vi "selfConfigRead.vi"(0 "RefDesType":string, 5 "error in":errorcluster) -> (14 "DAQ Node Array":string[](array[string]), 15 "DAQ Node Count":i32, 16 "refDes":string, 17 "IPaddr":string, 19 "error out":errorcluster)   [LabVIEW 2024]
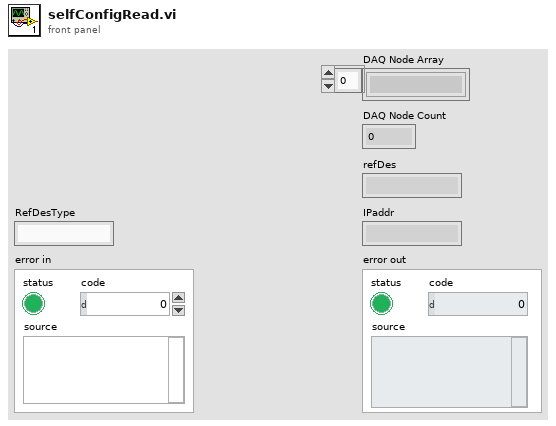
[diagram p1: front panel]
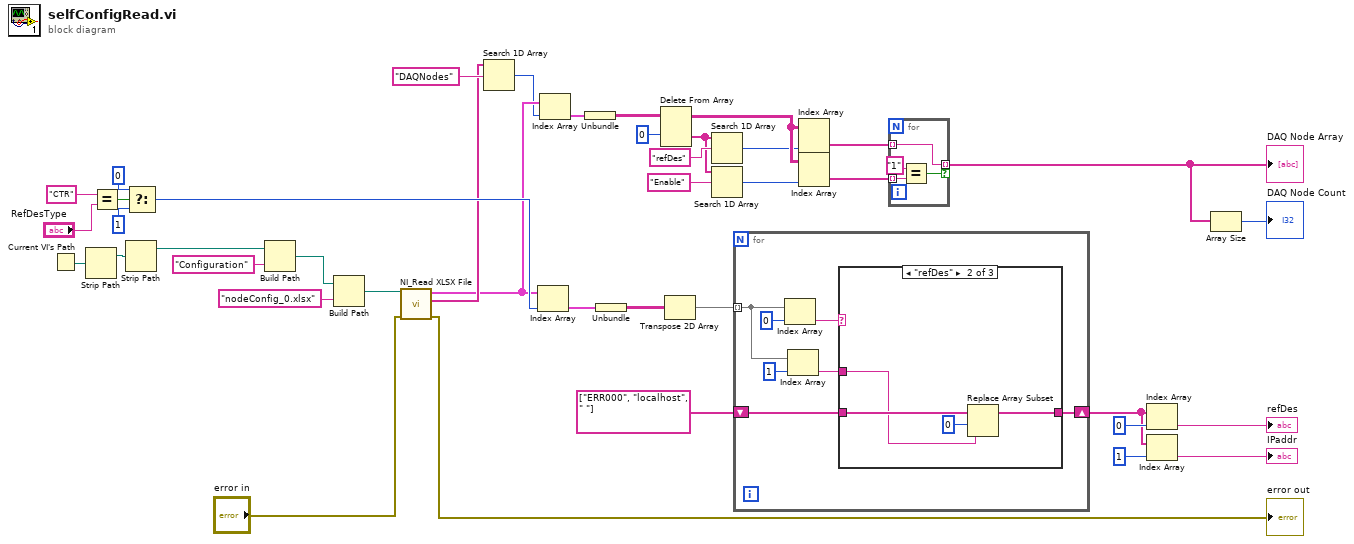
[diagram p0: block diagram]
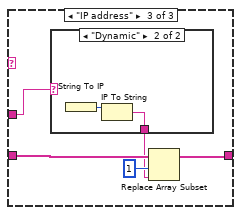
[diagram p3: hidden frame]
diagram:
  n1 = Current VI's Path() -> (path=w39:path)
  n2 = Strip Path(path=w39) -> (stripped path=w31:path)  [unwired: 1 out]
  n3 = Equal?(x="CTR", y="RefDesType") -> (x = y?=w27:bool)
  n4 = Strip Path(path=w31) -> (stripped path=w30:path)  [unwired: 1 out]
  n5 = Select(t=0, s=w27, f=1) -> (s? t:f=w24:i32)
  n6 = Build Path(base path=w30, name or relative path="Configuration") -> (appended path=w32:path)
  n7 = Build Path(base path=w32, name or relative path="nodeConfig_0.xlsx") -> (appended path=w40:path)
  n8 = call "NI_Read XLSX File.vi"("error in"="error in", "XLSX File"=w40) -> ("error out"=→"error out":errorcluster, "Sheet Names"=w16:string[], "Sheet Data"=w15:cluster{"Array":string[][]}[])  [unwired: 7 in]
  n9 = Search 1D Array(1D array=w16, element="DAQNodes") -> (index of element=w14:i32)  [unwired: 1 in]
  n10 = Index Array(array=w15, index=w24) -> (element=w23:cluster{"Array":string[][]})
  n11 = Index Array(array=w15, index=w14) -> (element=w13:cluster{"Array":string[][]})
  n12 = Unbundle(w13) -> ("Array"=w9:string[][])
  n13 = Unbundle(w23) -> ("Array"=w22:string[][])
  n14 = Delete From Array(array=w9, index (row)=0) -> (deleted portion=w8:string[], array with subset deleted=w7:string[][])  [unwired: 2 in]
  n15 = Transpose 2D Array(2D array=w22) -> (transposed array=w21:string[][])
  n16 = Search 1D Array(1D array=w8, element="refDes") -> (index of element=w5:i32)  [unwired: 1 in]
  n17 = Search 1D Array(1D array=w8, element="Enable") -> (index of element=w6:i32)  [unwired: 1 in]
  n18 = for {
    tunnel: w21 -> [w46] mode=indexing
    shift-right: [w43] -> w19
    shift-left: string[] ["ERR000", "localhost", " "] -> [w44]
    n19 = Index Array(array=w46, index=0) -> (element=w45:string)
    n20 = Index Array(array=w46, index=1) -> (element=w42:string)
    n21 = case shown="\"refDes\"" w45 {
      tunnel: w44 -> [w49 w53 w57]
      tunnel: [w49 w52 w56] -> w43
      tunnel: w42 -> [_ w50 w55]
      frame Default {
      }
      frame "refDes" {
        n22 = Replace Array Subset(array=w53, new element=w50, index=0) -> (w52:string[])
      }
      frame "IP address" {
        n23 = case shown="\"Dynamic\"" w55 {
          selector: w55 -> [w59 _]
          tunnel: [w59 w60] -> w54
          frame Default {
          }
          frame "Dynamic" {
            n24 = String To IP() -> (0:w61:u32)  [unwired: 1 in]
            n25 = IP To String(2:w61) -> (0:w60:string)  [unwired: 1 in]
          }
        }
        n26 = Replace Array Subset(array=w57, new element=w54, index=1) -> (w56:string[])
      }
    }
  }
  n27 = Index Array(array=w7, index (col)=w5) -> (element=w4:string[])  [unwired: 1 in]
  n28 = Index Array(array=w7, index (col)=w6) -> (element=w3:string[])  [unwired: 1 in]
  n29 = for {
    tunnel: w4 -> [w63] mode=indexing
    tunnel: w3 -> [w65] mode=indexing
    tunnel: [w63] -> w2 mode=indexing if=w62
    n30 = Equal?(x="1", y=w65) -> (x = y?=w62:bool)
  }
  "DAQ Node Array" <- w2
  n31 = Index Array(array=w19, index=0) -> (element=→"refDes":string)
  n32 = Index Array(array=w19, index=1) -> (element=→"IPaddr":string)
  n33 = Array Size(array=w2) -> (size(s)=→"DAQ Node Count":i32)
